vi "io.visa.vi"(6 "operation in (wr-rd)":T2=enum."IO_VISA_CLOSE", 7 "preReadMsDelay":u32=5, 8 "error in (no error)":errorcluster, 9 "Init Params":T1={"baud rate"=115200, "parity"=enum."None", "flow control"=0, "data bits"=8, "stop bits"=10, "timeout[ms]"=25, "Termination Char"="}", "End Read Mode"=2} {"baud rate" items=["75"=75, "110"=110, "134"=134, "150"=150, "300"=300, "600"=600, "1200"=1200, "1800"=1800, "2400"=2400, "4800"=4800, "7200"=7200, "9600"=9600, "14400"=14400, "19200"=19200, "28800"=28800, "38400"=38400, "56000"=56000, "57600"=57600, "115200"=115200, "128000"=128000, "230400"=230400]; "flow control" items=["None"=0, "XON/XOFF"=1, "RTS/CTS"=2, "DTR/DSR"=4]; "stop bits" items=["1.0"=10, "1.5"=15, "2.0"=20]; "End Read Mode" items=["None", "Last Bit", "TermChar"]}, 10 "write buffer":string, 11 "VISA Refnum in":refnum<visa-resource-name>) -> (0 "error out":errorcluster, 1 "delta":u32, 2 "read buffer":string, 3 "VISA Refnum out":refnum<visa-resource-name>="COM11")   [LabVIEW 2024]
uses:
  controls/enum.io-interface.ctl
  globals/globals-engine.vi
panel:
  out "return count":u32
  in  "postReadMsDelay":u32=1
  # "-1073807339\nVISA Read in io.visa.vi"
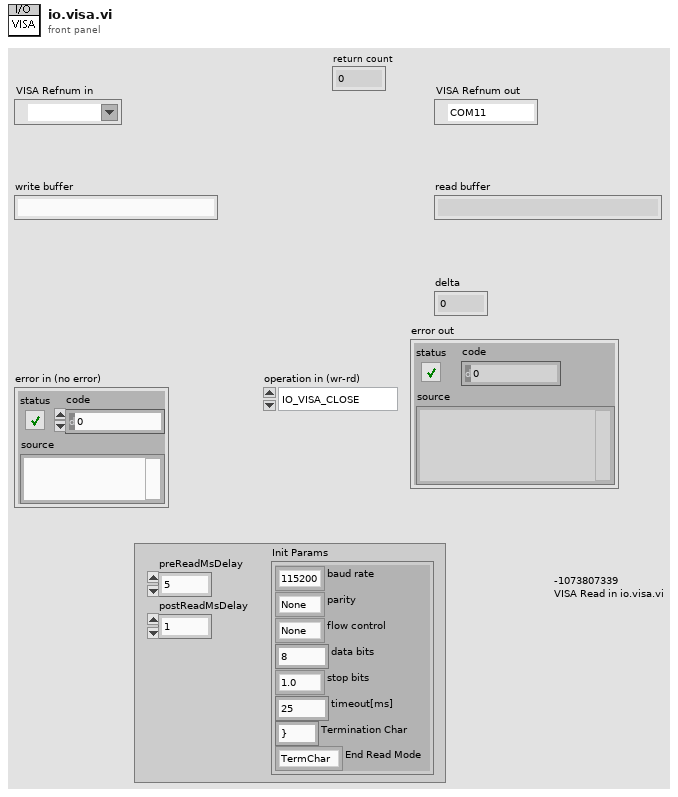
[diagram p1: front panel]
types:
  T1 = cluster{"baud rate":u32, "parity":enum16{"None", "Odd", "Even", "Mark", "Space"}, "flow control":u16, "data bits":u16, "stop bits":u16, "timeout[ms]":u32, "Termination Char":string, "End Read Mode":u16}
  T2 = typedef "enum.io-interface.ctl" = enum16{"IO_VISA_WR-RD", "IO_VISA_OPEN", "IO_VISA_CLOSE", "IO_VISA_CLEAR"}
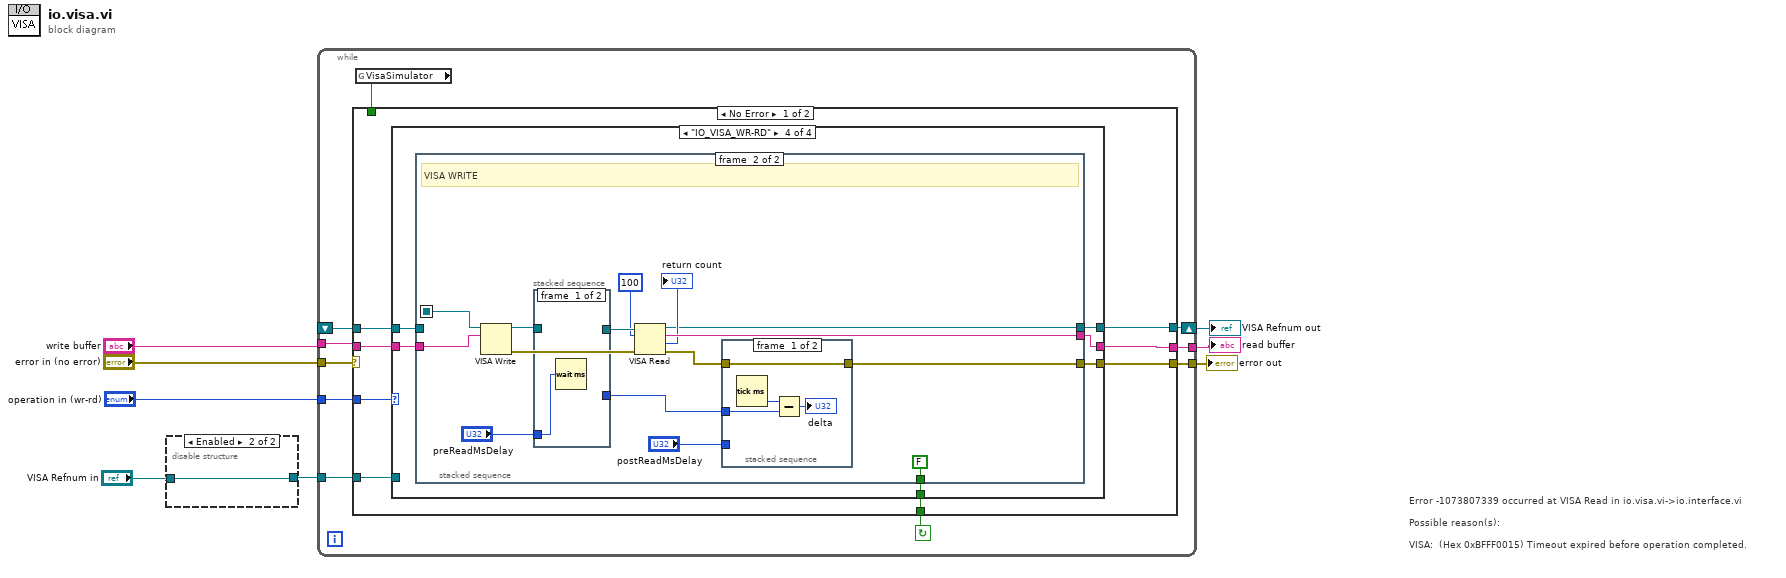
[diagram p0: block diagram]
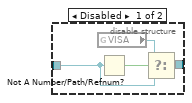
[diagram p2: hidden frame]
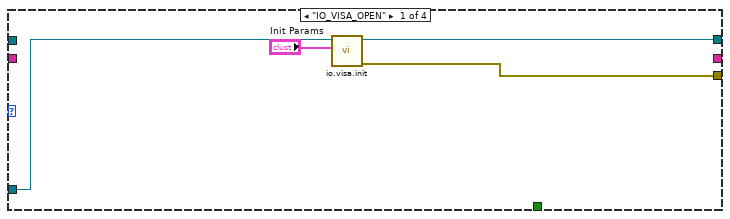
[diagram p3: hidden frame]
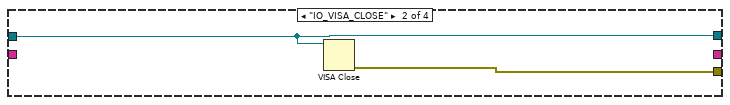
[diagram p4: hidden frame]
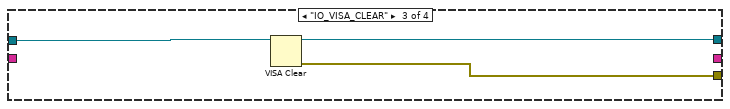
[diagram p5: hidden frame]
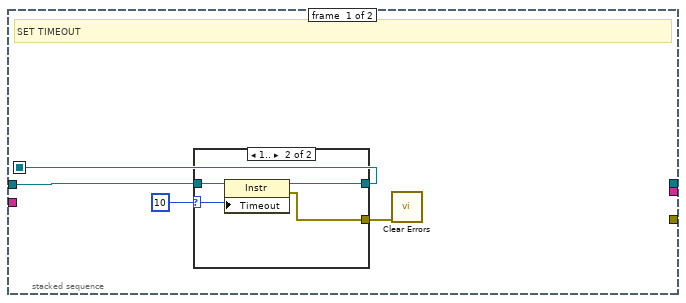
[diagram p6: hidden frame]
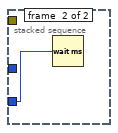
[diagram p8: hidden frame]
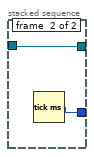
[diagram p9: hidden frame]
diagram:
  # "Error -1073807339 occurred at VISA Read in io.visa.vi->io.interface.vi\n\nPossible reason(s):\n\nVISA:  (Hex 0xBFFF0015) Timeout expired before operation completed."
  n1 = disable-structure shown="Enabled" {
    disable-tunnel: "VISA Refnum in" -> [w11 w13]
    disable-tunnel: [w9 w13] -> w1
    frame Disabled {
      n2 = global read "globals-engine.vi" "VISA"() -> (w10:refnum<visa-resource-name>)
      n3 = Not A Number/Path/Refnum?(number/path/refnum=w11) -> (NaN/Path/Refnum?=w12:bool)
      n4 = Select(t=w10, s=w12, f=w11) -> (s? t:f=w9:refnum<visa-resource-name>)
    }
    frame Enabled {
    }
  }
  n5 = while {
    tunnel: "operation in (wr-rd)" -> [w20]
    shift-right: [w22] -> w7
    shift-left: _ -> [w17]
    tunnel: "write buffer" -> [w21]
    tunnel: [w23] -> w8
    tunnel: "error in (no error)" -> [w18]
    tunnel: [w19] -> w4
    tunnel: w1 -> [w16]
    stop <- w14 continue-if-true
    n6 = global read "globals-engine.vi" "VisaSimulator"() -> (w15:bool)
    n7 = case shown="No Error" w18 {
      selector: w18 -> [_ w80]
      tunnel: [w31 _] -> w23
      tunnel: [w30 w79] -> w22
      tunnel: w17 -> [w29 w79]
      tunnel: w21 -> [w28 _]
      tunnel: w20 -> [w27 _]
      tunnel: [w26 w80] -> w19
      tunnel: w16 -> [w25 _]
      tunnel: w15 -> [_ _]
      tunnel: [w24 _] -> w14
      frame No Error {
        n8 = case shown="\"IO_VISA_WR-RD\"" w27 {
          tunnel: w28 -> [_ _ _ w46]
          tunnel: w29 -> [_ w37 w39 w42]
          tunnel: [w35 w37 w40 w45] -> w30
          tunnel: [_ _ _ w43] -> w31
          tunnel: [w33 w36 w38 w44] -> w26
          tunnel: w25 -> [w34 _ _ _]
          tunnel: [_ _ _ w41] -> w24
          frame "IO_VISA_OPEN" {
            n9 = call "io.visa.init.vi"("Init Params"="Init Params", "VISA Refnum in"=w34) -> ("error out"=w33:errorcluster, "VISA Refnum out"=w35:refnum<visa-resource-name>)  [unwired: 8 in]
          }
          frame "IO_VISA_CLOSE" {
            n10 = VISA Close(VISA resource name=w37) -> (error out=w36:errorcluster)  [unwired: 1 in]
          }
          frame "IO_VISA_CLEAR" {
            n11 = VISA Clear(VISA resource name=w39) -> (VISA resource name out=w40:refnum<visa-resource-name>, error out=w38:errorcluster)  [unwired: 1 in]
          }
          frame "IO_VISA_WR-RD" {
            n12 = stacked-sequence {
              seq-local: [w49 _] -> [_ w67]
              tunnel: w46 -> [_ w70]
              tunnel: [_ w56] -> w45
              tunnel: [_ w58] -> w44
              tunnel: [_ w69] -> w43
              tunnel: w42 -> [w50 _]
              tunnel: [_ FALSE] -> w41
              frame #0 {
                # "SET TIMEOUT"
                n13 = case shown="1.." u32 10 ("ReadTimeout") {
                  selector: u32 10 ("ReadTimeout") -> [_ w53]
                  tunnel: w50 -> [w51 w55]
                  tunnel: [w51 w54] -> w49
                  tunnel: [_ w52] -> w47
                  frame Default {
                  }
                  frame 1.. {
                    n14 = property class="Instr"(reference=w55, "Timeout"=w53) -> (reference out=w54:refnum<visa-resource-name>, error out=w52:errorcluster)  [unwired: 1 in]
                  }
                }
                n15 = call <vilib>:"Clear Errors.vi"("error in (no error)"=w47) -> ()  [unwired: 5 in, 2 out]
              }
              frame #1 {
                # "VISA WRITE"
                n16 = VISA Write(VISA resource name=w67, write buffer=w70) -> (VISA resource name out=w64:refnum<visa-resource-name>, error out=w66:errorcluster)  [unwired: 1 in, 1 out]
                n17 = stacked-sequence {
                  tunnel: [_ w78] -> w65
                  tunnel: w64 -> [_ w78]
                  tunnel: [_ w77] -> w61
                  tunnel: "preReadMsDelay" -> [w76 _]
                  frame #0 {
                    n18 = Wait (ms)(milliseconds to wait=w76) -> ()  [unwired: 1 out]
                  }
                  frame #1 {
                    n19 = Tick Count (ms)() -> (millisecond timer value=w77:u32)
                  }
                }
                n20 = VISA Read(VISA resource name=w65, byte count=u32 100, error in (no error)=w66) -> (VISA resource name out=w56:refnum<visa-resource-name>, read buffer=w69:string, return count=→"return count":u32, error out=w62:errorcluster)
                n21 = stacked-sequence {
                  tunnel: [w74 _] -> w58
                  tunnel: w62 -> [w74 _]
                  tunnel: w61 -> [w72 _]
                  tunnel: "postReadMsDelay" -> [_ w75]
                  frame #0 {
                    n22 = Tick Count (ms)() -> (millisecond timer value=w73:u32)
                    n23 = Subtract(x=w73, y=w72) -> (x-y=→"delta":u32)
                  }
                  frame #1 {
                    n24 = Wait (ms)(milliseconds to wait=w75) -> ()  [unwired: 1 out]
                  }
                }
              }
            }
          }
        }
      }
      frame Error {
      }
    }
  }
  "read buffer" <- w8
  "VISA Refnum out" <- w7
  "error out" <- w4
